vi "Main.vi"(11 "Module Admin":refnum<class "Delacor_lib_QMH_Module Admin.lvclass">) -> ()   [LabVIEW 2018, in "Example.lvlib"]
doc: "This template is based off of the Queued Message Handler design pattern and the Queued Message Handler project template that ships with LabVIEW.\n\nThe main difference is that the queue is private to this module and communication between modules is performed via Broadcast and Request events.\n\nRequest events are wrapped in public API methods and are handled in the Event Handling Loop (EHL) of this VI. Any module can register for Broadcast events sent by this module. The EHL generates messages based on user interface actions.\n\nThe Message Handling Loop (MHL) processes messages generated by the EHL, or by other messages. The messages are string values, so new messages can be added easily to the Message Cases case structure in the MHL. Each message cluster can also provide an optional value for Message Data, which is a variant that can be converted to whatever message-specific data is required.\n_____\nBased on DQMH Project Example 6.0.0.91."
uses:
  Example.lvlib
  <vilib>/Delacor/Delacor QMH/Libraries/Message Queue_class/Delacor_lib_QMH_Message Queue.lvclass
  Module Data--cluster.ctl
  <vilib>/Utility/miscctls.llb/LVPointTypeDef.ctl
  Do Something Argument--cluster.ctl
  Do Something Else Argument--cluster.ctl
  Do Something Else and Wait (Reply Payload)--cluster.ctl
  Do Something Else and Wait for Reply Argument--cluster.ctl
  <vilib>/Utility/error.llb/Error Cluster From Error Code.vi
  <vilib>/ErrorRing/Error Ring.xnode
  <vilib>/Delacor/Delacor QMH/Libraries/Message Queue_class/Delacor_lib_QMH_Enqueue Message (Single).vi
  Stop Argument--cluster.ctl
  <vilib>/Delacor/Delacor QMH/Libraries/Module Admin_class/Delacor_lib_QMH_Module Admin.lvclass
  Get Bitness Info (Reply Payload)--cluster.ctl
  Get Bitness Info Argument--cluster.ctl
panel:
  out "error out":errorcluster
  out "X":dbl
  out "Status":string
  in  "Simulate MHL Error":bool
  in  "Simulate EHL Error":bool
  in  "Do Something Else <Replace Me>":bool
  in  "Do Something <Replace Me>":bool
  # "These controls have associated \"Value Changed\" events configured in the Event Structure on the diagram.\n\nReplace them (and reconfigure the Event Structure) with the controls you need for your application. \n\nOther QMH Modules communicate with this Module via its Public API (wrappers for its Request Events).\n\nThis Module communicates with other Modules via its Broadcast Events.\nAny module that wants to get these messages, just registers for this module's Broadcast events."
  # "This template is for the Delacor Modified Queued Message Handler design pattern.\n\nSee the block diagram for more information on how to use this template."
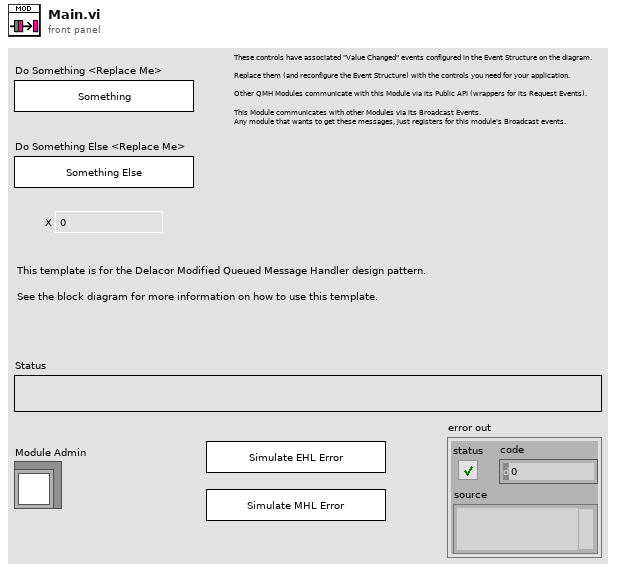
[diagram p1: front panel]
types:
  T1 = typedef "Example.lvlib/Request Events--cluster.ctl" = cluster{"Stop Module":refnum<user-event>, "Do Something":refnum<user-event>, "Do Something Else":refnum<user-event>, "Do Something Else and Wait for Reply":refnum<user-event>, "Show Panel":refnum<user-event>, "Hide Panel":refnum<user-event>, "Get Module Execution Status":refnum<user-event>, "Show Diagram":refnum<user-event>, "Get Bitness Info":refnum<user-event>}
  T2 = typedef "Example.lvlib/Module Data--cluster.ctl" = cluster{"Status":string}
  T3 = typedef "Example.lvlib/Do Something Argument--cluster.ctl" = cluster{"Do Something Msg":string}
  T4 = typedef "Example.lvlib/Do Something Else Argument--cluster.ctl" = cluster{"Do Something Else Msg":string, "X":dbl}
  T5 = typedef "Example.lvlib/Do Something Else and Wait for Reply Argument--cluster.ctl" = cluster{"Do Something Else Msg":string, "X":dbl, "Wait Notifier":refnum<notifier>, "wait for reply":bool}
  T6 = enum32{"invalid lock state", "Not Locked", "Locked (No Password)", "Password-protected"}
  T7 = typedef "Example.lvlib/Stop Argument--cluster.ctl" = cluster{"Origin":string, "Exit via Stop Module Req?":bool, "Wait for Module to stop?":bool}
  T8 = typedef "Example.lvlib/Get Bitness Info Argument--cluster.ctl" = cluster{"Wait Notifier":refnum<notifier>, "wait for reply":bool}
  T9 = typedef "LVPointTypeDef.ctl" = cluster{"Horizontal":i16, "Vertical":i16}
  T10 = enum32{"Invalid", "Standard", "Closed", "Hidden", "Minimized", "Maximized"}
  T11 = typedef "Example.lvlib/Do Something Else and Wait (Reply Payload)--cluster.ctl" = cluster{"Value":dbl, "error":errorcluster}
  T12 = typedef "Example.lvlib/Get Bitness Info (Reply Payload)--cluster.ctl" = cluster{"BitnessInfo":string, "Get Bitness Info_error":errorcluster}
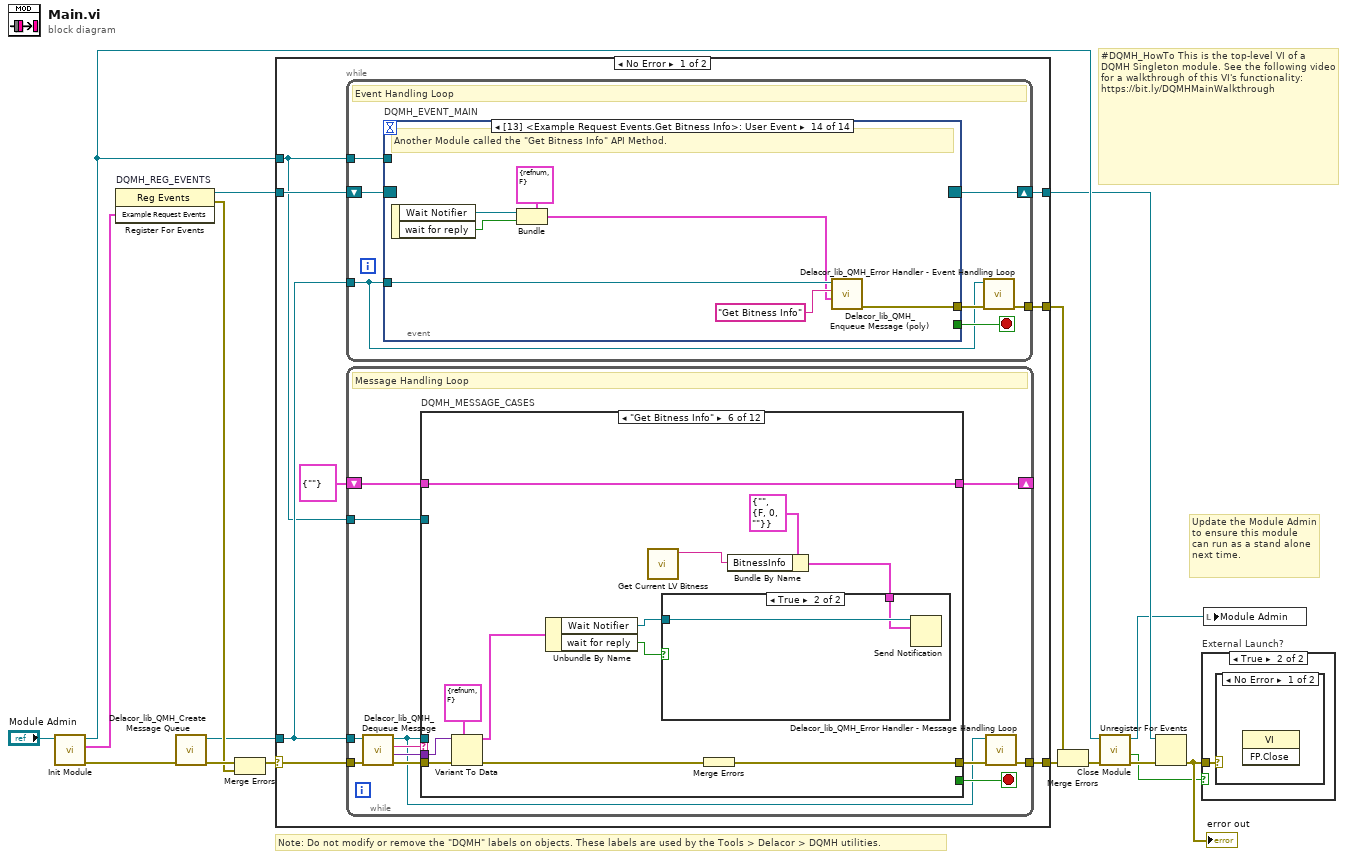
[diagram p0: block diagram]
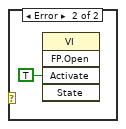
[diagram p3: hidden frame]
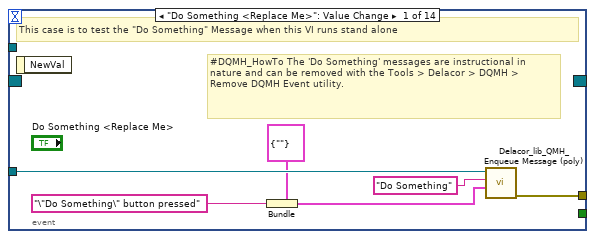
[diagram p4: hidden frame]
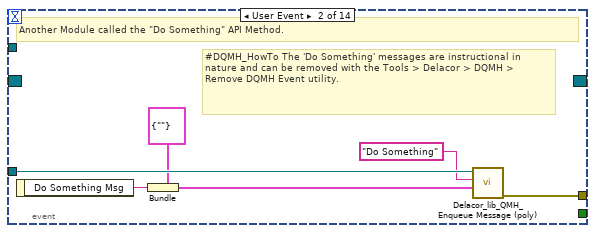
[diagram p5: hidden frame]
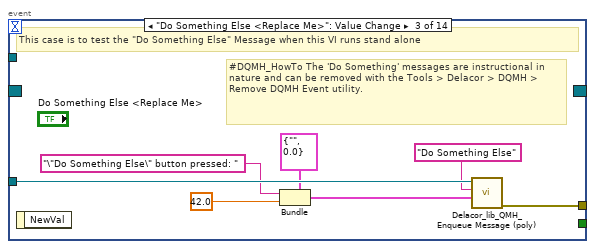
[diagram p6: hidden frame]
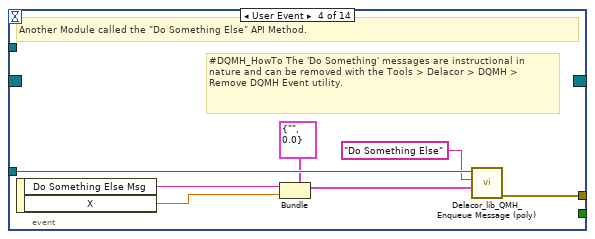
[diagram p7: hidden frame]
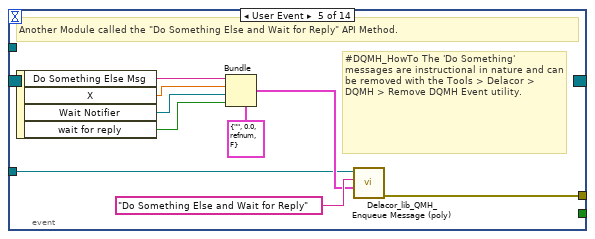
[diagram p8: hidden frame]
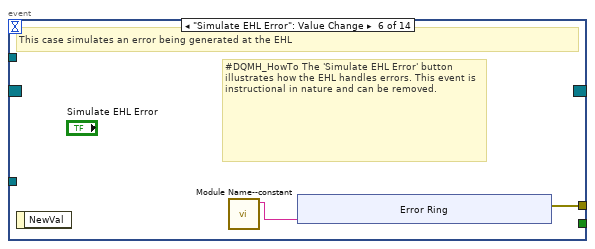
[diagram p9: hidden frame]
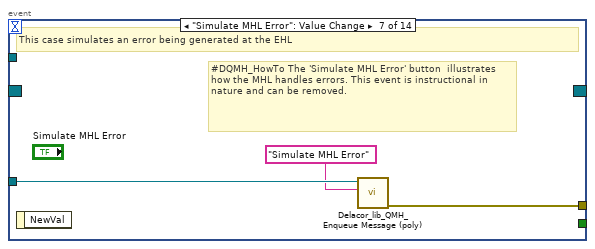
[diagram p10: hidden frame]
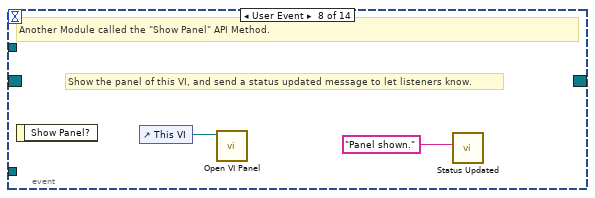
[diagram p11: hidden frame]
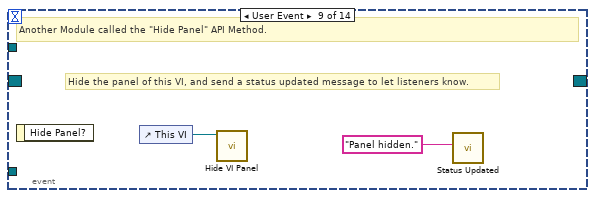
[diagram p12: hidden frame]
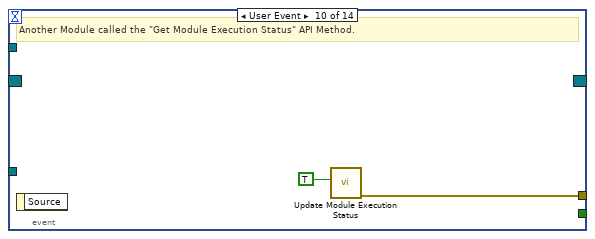
[diagram p13: hidden frame]
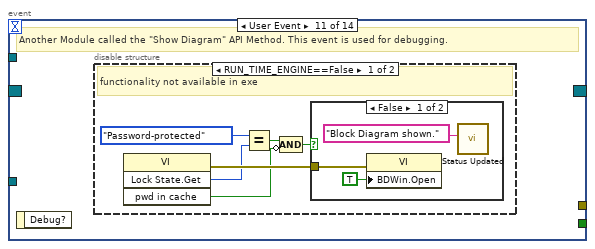
[diagram p14: hidden frame]
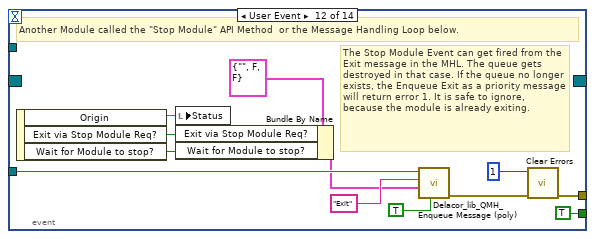
[diagram p17: hidden frame]
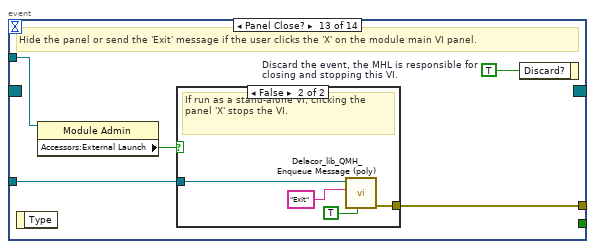
[diagram p18: hidden frame]
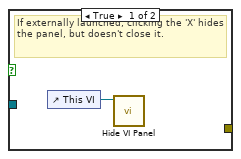
[diagram p19: hidden frame]
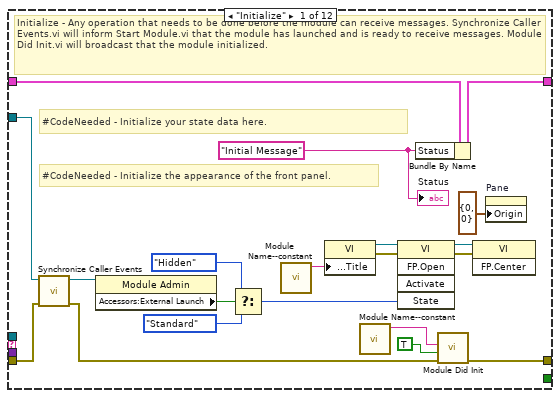
[diagram p20: hidden frame]
diagram:
  # "#DQMH_HowTo This is the top-level VI of a DQMH Singleton module. See the following video for a walkthrough of this VI's functionality: https://bit.ly/DQMHMainWalkthrough"
  # "Note: Do not modify or remove the \"DQMH\" labels on objects. These labels are used by the Tools > Delacor > DQMH utilities."
  # "Update the Module Admin to ensure this module can run as a stand alone next time."
  n1 = call "Init Module.vi"("Singleton Module Admin in"="Module Admin") -> ("error out"=w16:errorcluster, "Example Request Events"=w5:T1, "Singleton Module Admin out"=w8:refnum<class "Delacor_lib_QMH_Module Admin.lvclass">)  [unwired: 8 in]
  n2 = register-events "DQMH_REG_EVENTS"(w5) -> (reference out=w6:refnum<event-registration>, error out=w9:errorcluster)  [unwired: 2 in]
  n3 = call <vilib>:"Delacor_lib_QMH_Create Message Queue.vi"("error in"=w16) -> ("error out"=w11:errorcluster, "Message Queue"=w4:refnum<class "Delacor_lib_QMH_Message Queue.lvclass">)  [unwired: 9 in]
  n4 = Merge Errors(w11, w9) -> (w10:errorcluster)
  n5 = case shown="No Error" w10 {
    selector: w10 -> [w23 w284]
    tunnel: [w25 w283] -> w17
    tunnel: [w22 w289] -> w7
    tunnel: w6 -> [w20 w289]
    tunnel: w4 -> [w19 w282]
    tunnel: [w24 _] -> w14
    tunnel: w8 -> [w18 w285]
    frame No Error {
      n6 = while {
        tunnel: w19 -> [w26]
        shift-right: [w29] -> w22
        shift-left: w20 -> [w30]
        tunnel: [w31] -> w24
        tunnel: w18 -> [w27]
        stop <- w28 stop-if-true
        # "Event Handling Loop"
        n7 = event "DQMH_EVENT_MAIN" shown="[13] <Example Request Events.Get Bitness Info>: User Event" {
          selector: w30 -> [_ _ _ _ _ _ _ _ _ _ _ _ _ _]
          dyn-events: [_ _ _ _ _ _ _ _ _ _ _ _ _ _] -> w29
          timeout: _ -> [_ _ _ _ _ _ _ _ _ _ _ _ _ _]
          tunnel: [_ _ _ _ _ _ _ _ _ _ _ TRUE ("Discard?") _ _] -> w28
          tunnel: w26 -> [w37 w43 w50 w57 w60 _ w78 _ _ _ _ w102 w109 w123]
          tunnel: [w38 w44 w51 w58 w67 w69 w79 _ _ w85 _ w105 w111 w117] -> w32
          tunnel: w27 -> [_ _ _ _ _ _ _ _ _ _ _ _ w108 _]
          event "Do Something <Replace Me>": Value Change {
            # "#DQMH_HowTo The 'Do Something' messages are instructional in nature and can be removed with the Tools > Delacor > DQMH > Remove DQMH Event utility."
            # "This case is to test the \"Do Something\" Message when this VI runs stand alone"
            n8 = event-data() -> ()  [unwired: 1 in, 1 out]
            n9 = Bundle(cluster=T3 {"Do Something Msg"=""} ("Do Something Argument"), "Do Something Msg"="\"Do Something\" button pressed" ("\"Do Something\" button pressed")) -> (w33:T3)
            n10 = call-poly <vilib>:"Delacor_lib_QMH_Enqueue Message (poly).vi"("Message Data"=w33, "Message"="Do Something", "Message Queue in"=w37) -> ("error out"=w38:errorcluster)  [unwired: 7 in, 1 out]
          }
          event User Event {
            # "#DQMH_HowTo The 'Do Something' messages are instructional in nature and can be removed with the Tools > Delacor > DQMH > Remove DQMH Event utility."
            # "Another Module called the \"Do Something\" API Method."
            n11 = event-data() -> ("Do Something Msg"=w40:string)  [unwired: 1 in]
            n12 = Bundle(cluster=T3 {"Do Something Msg"=""} ("Do Something Argument"), "Do Something Msg"=w40) -> (w39:T3)
            n13 = call-poly <vilib>:"Delacor_lib_QMH_Enqueue Message (poly).vi"("Message Data"=w39, "Message"="Do Something", "Message Queue in"=w43) -> ("error out"=w44:errorcluster)  [unwired: 7 in, 1 out]
          }
          event "Do Something Else <Replace Me>": Value Change {
            # "#DQMH_HowTo The 'Do Something' messages are instructional in nature and can be removed with the Tools > Delacor > DQMH > Remove DQMH Event utility."
            # "This case is to test the \"Do Something Else\" Message when this VI runs stand alone"
            n14 = event-data() -> ()  [unwired: 1 in, 1 out]
            n15 = Bundle(cluster=T4 {"Do Something Else Msg"="", "X"=0.0} ("Do Something Else Argument"), "Do Something Else Msg"="\"Do Something Else\" button pressed: " ("\"Do Something Else\" button pressed"), "X"=42.0) -> (w47:T4)
            n16 = call-poly <vilib>:"Delacor_lib_QMH_Enqueue Message (poly).vi"("Message Data"=w47, "Message"="Do Something Else", "Message Queue in"=w50) -> ("error out"=w51:errorcluster)  [unwired: 7 in, 1 out]
          }
          event User Event {
            # "#DQMH_HowTo The 'Do Something' messages are instructional in nature and can be removed with the Tools > Delacor > DQMH > Remove DQMH Event utility."
            # "Another Module called the \"Do Something Else\" API Method."
            n17 = event-data() -> ("Do Something Else Msg"=w53:string, "X"=w52:dbl)  [unwired: 1 in]
            n18 = Bundle(cluster=T4 {"Do Something Else Msg"="", "X"=0.0} ("Do Something Else Argument"), "Do Something Else Msg"=w53, "X"=w52) -> (w54:T4)
            n19 = call-poly <vilib>:"Delacor_lib_QMH_Enqueue Message (poly).vi"("Message Data"=w54, "Message"="Do Something Else", "Message Queue in"=w57) -> ("error out"=w58:errorcluster)  [unwired: 7 in, 1 out]
          }
          event User Event {
            # "#DQMH_HowTo The 'Do Something' messages are instructional in nature and can be removed with the Tools > Delacor > DQMH > Remove DQMH Event utility."
            # "Another Module called the \"Do Something Else and Wait for Reply\" API Method."
            n20 = event-data() -> ("Do Something Else Msg"=w63:string, "X"=w62:dbl, "Wait Notifier"=w61:refnum<notifier>, "wait for reply"=w59:bool)  [unwired: 1 in]
            n21 = Bundle(cluster=T5 {"Do Something Else Msg"="", "X"=0.0, "Wait Notifier"=refnum, "wait for reply"=FALSE} ("Do Something Else and Wait for Reply Argument"), "Do Something Else Msg"=w63, "X"=w62, "Wait Notifier"=w61, "wait for reply"=w59) -> (w64:T5)
            n22 = call-poly <vilib>:"Delacor_lib_QMH_Enqueue Message (poly).vi"("Message Data"=w64, "Message"="Do Something Else and Wait for Reply", "Message Queue in"=w60) -> ("error out"=w67:errorcluster)  [unwired: 7 in, 1 out]
          }
          event "Simulate EHL Error": Value Change {
            # "#DQMH_HowTo The 'Simulate EHL Error' button  illustrates how the EHL handles errors. This event is instructional in nature and can be removed."
            # "This case simulates an error being generated at the EHL"
            n23 = event-data() -> ()  [unwired: 1 in, 1 out]
            n24 = call "Module Name--constant.vi"() -> ("Module Name"=w68:string)  [unwired: 11 in]
            n25 = xnode "Error Ring"("parameter 0"=w68) -> ("error out"=w69:errorcluster)
          }
          event "Simulate MHL Error": Value Change {
            # "#DQMH_HowTo The 'Simulate MHL Error' button  illustrates how the MHL handles errors. This event is instructional in nature and can be removed."
            # "This case simulates an error being generated at the EHL"
            n26 = event-data() -> ()  [unwired: 1 in, 1 out]
            n27 = call-poly <vilib>:"Delacor_lib_QMH_Enqueue Message (poly).vi"("Message"="Simulate MHL Error", "Message Queue in"=w78) -> ("error out"=w79:errorcluster)  [unwired: 8 in, 1 out]
          }
          event User Event {
            # "Show the panel of this VI, and send a status updated message to let listeners know."
            # "Another Module called the \"Show Panel\" API Method."
            n28 = event-data() -> ()  [unwired: 1 in, 1 out]
            n29 = control-ref of="This VI"() -> (w81:refnum<vi>)
            n30 = call "Open VI Panel.vi"("VI"=w81) -> ()  [unwired: 10 in, 1 out]
            n31 = call "Status Updated.vi"("Status"="Panel shown." ("format string")) -> ()  [unwired: 10 in, 1 out]
          }
          event User Event {
            # "Hide the panel of this VI, and send a status updated message to let listeners know."
            # "Another Module called the \"Hide Panel\" API Method."
            n32 = event-data() -> ()  [unwired: 1 in, 1 out]
            n33 = control-ref of="This VI"() -> (w83:refnum<vi>)
            n34 = call "Hide VI Panel.vi"("VI"=w83) -> ()  [unwired: 10 in, 1 out]
            n35 = call "Status Updated.vi"("Status"="Panel hidden." ("format string")) -> ()  [unwired: 10 in, 1 out]
          }
          event User Event {
            # "Another Module called the \"Get Module Execution Status\" API Method."
            n36 = event-data() -> ()  [unwired: 1 in, 1 out]
            n37 = call "Update Module Execution Status.vi"("Running?"=TRUE) -> ("error out"=w85:errorcluster)  [unwired: 10 in]
          }
          event User Event {
            # "Another Module called the \"Show Diagram\" API Method. This event is used for debugging."
            n38 = event-data() -> ()  [unwired: 1 in, 1 out]
            n39 = disable-structure shown="RUN_TIME_ENGINE==False" {
              frame condition #0 (active) {
                # "functionality not available in exe"
                n40 = invoke class="VI" method="Lock State.Get"() -> (error out=w91:errorcluster, "Get Lock State"=w90:T6, "pwd in cache"=w87:bool)  [unwired: 4 in, 1 out]
                n41 = Equal?(x=T6."Password-protected", y=w90) -> (x = y?=w88:bool)
                n42 = Compound Arithmetic op=AND(w88, invert w87) -> (w86:bool)
                n43 = case shown="False" w86 {
                  tunnel: w91 -> [w94 _]
                  frame False {
                    n44 = property class="VI"(error in=w94, "BDWin.Open"=TRUE ("Block Diagram Window:Open")) -> ()  [unwired: 1 in, 2 out]
                    n45 = call "Status Updated.vi"("Status"="Block Diagram shown." ("format string")) -> ()  [unwired: 10 in, 1 out]
                  }
                  frame True {
                    # "Password-protected VI, and the password is not in the cache. Do not show the diagram."
                  }
                }
              }
              frame condition #1 {
              }
            }
          }
          event User Event {
            # "The Stop Module Event can get fired from the Exit message in the MHL. The queue gets destroyed in that case. If the queue no longer exists, the Enqueue Exit as a priority message will return error 1. It is safe to ignore, because the module is already exiting."
            # "Another Module called the \"Stop Module\" API Method  or the Message Handling Loop below."
            n46 = event-data() -> ("Origin"=w101:string, "Exit via Stop Module Req?"=w97:bool, "Wait for Module to stop?"=w96:bool)  [unwired: 1 in]
            n47 = local write "Status"(w101) -> ()
            n48 = Bundle By Name(cluster=T7 {"Origin"="", "Exit via Stop Module Req?"=FALSE, "Wait for Module to stop?"=FALSE} ("Stop Argument"), "Exit via Stop Module Req?"=w97, "Wait for Module to stop?"=w96) -> (w95:T7)
            n49 = call-poly <vilib>:"Delacor_lib_QMH_Enqueue Message (poly).vi"("Priority Message? (F)"=TRUE, "Message Data"=w95, "Message"="Exit", "Message Queue in"=w102) -> ("error out"=w106:errorcluster)  [unwired: 6 in, 1 out]
            n50 = call <vilib>:"Clear Errors.vi"("error in (no error)"=w106, "specific error code to clear (0: all)"=1) -> ("error out"=w105:errorcluster)  [unwired: 4 in, 1 out]
          }
          event Panel Close? {
            w110 = TRUE  # Discard the event, the MHL is responsible for closing and stopping this VI.
            # "Hide the panel or send the 'Exit' message if the user clicks the 'X' on the module main VI panel."
            n51 = event-data() -> ()  [unwired: 1 in, 1 out]
            n52 = property class="Module Admin"(reference=w108) -> ("Accessors:External Launch"=w107:bool)  [unwired: 1 in, 2 out]
            n53 = case shown="False" w107 {
              tunnel: w109 -> [_ w115]
              tunnel: [_ w116] -> w111
              frame True {
                # "If externally launched, clicking the 'X' hides the panel, but doesn't close it."
                n54 = control-ref of="This VI"() -> (w112:refnum<vi>)
                n55 = call "Hide VI Panel.vi"("VI"=w112) -> ()  [unwired: 10 in, 1 out]
              }
              frame False {
                # "If run as a stand-alone VI, clicking the panel 'X' stops the VI."
                n56 = call-poly <vilib>:"Delacor_lib_QMH_Enqueue Message (poly).vi"("Priority Message? (F)"=TRUE, "Message"="Exit", "Message Queue in"=w115) -> ("error out"=w116:errorcluster)  [unwired: 7 in, 1 out]
              }
            }
            n57 = event-data("Discard?"=w110) -> ()  [unwired: 1 in, 1 out]
          }
          event User Event {
            # "Another Module called the \"Get Bitness Info\" API Method."
            n58 = event-data() -> ("Wait Notifier"=w119:refnum<notifier>, "wait for reply"=w118:bool)  [unwired: 1 in]
            n59 = Bundle(cluster=T8 {"Wait Notifier"=refnum, "wait for reply"=FALSE} ("Get Bitness Info Argument"), "Wait Notifier"=w119, "wait for reply"=w118) -> (w120:T8)
            n60 = call-poly <vilib>:"Delacor_lib_QMH_Enqueue Message (poly).vi"("Message Data"=w120, "Message"="Get Bitness Info", "Message Queue in"=w123) -> ("error out"=w117:errorcluster)  [unwired: 7 in, 1 out]
          }
        }
        n61 = call-dynamic "Delacor_lib_QMH_Error Handler - Event Handling Loop.vi"("error in"=w32, "Message Queue in"=w26) -> ("dup error in"=w31:errorcluster)  [unwired: 8 in, 1 out]
      }
      n62 = while {
        tunnel: w19 -> [w126]
        shift-right: [w130] -> _
        shift-left: T2 {"Status"=""} ("Data Cluster") -> [w131]
        tunnel: w23 -> [w134]
        tunnel: [w132] -> w25
        tunnel: w18 -> [w124]
        stop <- w129 stop-if-true
        # "Message Handling Loop"
        n63 = call-dynamic "Delacor_lib_QMH_Dequeue Message.vi"("error in"=w134, "Message Queue in"=w126) -> ("error out"=w133:errorcluster, "Message Data"=w127:variant, "Message"=w128:string, "Message Queue out"=w125:refnum<class "Delacor_lib_QMH_Message Queue.lvclass">)  [unwired: 6 in]
        n64 = case "DQMH_MESSAGE_CASES" shown="\"Get Bitness Info\"" w128 {
          selector: w128 -> [_ _ _ _ _ _ _ _ _ _ _ w269]
          tunnel: w125 -> [_ _ _ _ _ _ _ _ _ w239 w261 _]
          tunnel: w133 -> [w153 w157 w165 w174 w193 w217 w222 w224 w229 w246 w267 w271]
          tunnel: [w151 w157 w163 w173 w192 w207 w221 w224 w228 w242 w264 w272] -> w135
          tunnel: w131 -> [w142 w156 w162 w172 w190 w216 w220 w223 w226 w241 w260 w270]
          tunnel: [w141 w156 w162 w172 w190 w216 w220 w223 w226 w241 w260 w270] -> w130
          tunnel: [_ _ _ _ _ _ _ _ _ _ w259 _] -> w129
          tunnel: w127 -> [_ _ w161 w169 w187 w214 _ _ _ w240 w258 _]
          tunnel: w124 -> [w143 _ _ _ _ _ _ _ _ w238 w253 _]
          frame "Initialize" {
            w137 = "Initial Message" ("Initial Message")
            # "#CodeNeeded - Initialize the appearance of the front panel."
            # "#CodeNeeded - Initialize your state data here."
            # "Initialize - Any operation that needs to be done before the module can receive messages. Synchronize Caller Events.vi will inform Start Module.vi that the module has launched and is ready to receive messages. Module Did Init.vi will broadcast that the module initialized."
            n65 = call "Synchronize Caller Events.vi"("error in (no error)"=w153, "Singleton Module Admin in"=w143) -> ("error out"=w152:errorcluster, "Singleton Module Admin out"=w138:refnum<class "Delacor_lib_QMH_Module Admin.lvclass">)  [unwired: 8 in]
            n66 = property class="Module Admin"(reference=w138) -> ("Accessors:External Launch"=w147:bool)  [unwired: 1 in, 2 out]
            n67 = Select(t=T10."Hidden" ("State"), s=w147, f=T10."Standard" ("State")) -> (s? t:f=w144:T10)
            n68 = call "Module Name--constant.vi"() -> ("Module Name"=w150:string)  [unwired: 11 in]
            n69 = property class="VI"("Front Panel.Title"=w150) -> (reference out=w149:refnum<vi>, error out=w155:errorcluster)  [unwired: 2 in]
            n70 = call "Module Name--constant.vi"() -> ("Module Name"=w139:string)  [unwired: 11 in]
            n71 = invoke class="VI" method="FP.Open"(reference=w149, error in=w155, "State"=w144) -> (reference out=w148:refnum<vi>, error out=w154:errorcluster)  [unwired: 2 in, 3 out]
            n72 = Bundle By Name(cluster=w142, "Status"=w137) -> (w141:T2)
            n73 = call "Module Did Init.vi"("error in (no error)"=w152, "Initialized?"=TRUE, "Origin"=w139) -> ("error out"=w151:errorcluster)  [unwired: 8 in]
            n74 = invoke class="VI" method="FP.Center"(reference=w148, error in=w154) -> ()  [unwired: 1 in, 3 out]
            n75 = property on="Pane" class="Pane"("Origin"=T9 {"Horizontal"=0, "Vertical"=0}) -> ()  [unwired: 2 in, 2 out]
            "Status" <- w137
          }
          frame "---Module Specific---" {
            # "Separator -- The following cases handle messages specific to this Module."
          }
          frame "Do Something" {
            # "#DQMH_HowTo The 'Do Something' messages are instructional in nature and can be removed with the Tools > Delacor > DQMH > Remove DQMH Event utility."
            # "Do Something - Replace this message with functionality for your own application. Note that this message also fires the \"Did Something\" broadcast event."
            n76 = Variant To Data(error in=w165, type=T3 {"Do Something Msg"=""} ("Do Something Argument"), Variant=w161) -> (data=w160:T3, error out=w164:errorcluster)
            n77 = Unbundle By Name(w160) -> ("Do Something Msg"=w158:string)
            n78 = call "Did Something.vi"("error in (no error)"=w164, "Did Something Msg"=w158) -> ("error out"=w163:errorcluster)  [unwired: 9 in]
            n79 = local write "Status"(w158) -> ()
            n80 = call "Status Updated.vi"("Status"=w158) -> ()  [unwired: 10 in, 1 out]
          }
          frame "Do Something Else" {
            # "#DQMH_HowTo The 'Do Something' messages are instructional in nature and can be removed with the Tools > Delacor > DQMH > Remove DQMH Event utility."
            # "Do Something Else - Replace this message with functionality for your own application."
            n81 = Variant To Data(error in=w174, type=T4 {"Do Something Else Msg"="", "X"=0.0} ("Do Something Else Argument"), Variant=w169) -> (data=w170:T4, error out=w173:errorcluster)
            n82 = Unbundle By Name(w170) -> ("Do Something Else Msg"=w168:string, "X"=w167:dbl)
            "X" <- w167
            n83 = Format Into String(initial string=w168, w167) -> (resulting string=w166:string)  [unwired: 2 in, 1 out]
            n84 = local write "Status"(w166) -> ()
            n85 = call "Status Updated.vi"("Status"=w166) -> ()  [unwired: 10 in, 1 out]
          }
          frame "Do Something Else and Wait for Reply" {
            w182 = "X(%.2f)+Offset(%.2f)=%.2f"  # status message format string
            # "#DQMH_HowTo The 'Do Something' messages are instructional in nature and can be removed."
            # "Send back X with a random offset"
            # "Do Something Else and Wait for Reply - Replace this message with functionality for your own application. Note that this message must fire a notifier to let callers know it has finished execution, and it returns an error if the 'Value' is negative."
            n86 = Random Number (0-1)() -> (number: 0 to 1=w184:dbl)
            n87 = Variant To Data(error in=w193, type=T5 {"Do Something Else Msg"="", "X"=0.0, "Wait Notifier"=refnum, "wait for reply"=FALSE} ("Do Something Else and Wait for Reply Argument"), Variant=w187) -> (data=w188:T5, error out=w191:errorcluster)
            n88 = Unbundle By Name(w188) -> ("Wait Notifier"=w175:refnum<notifier>, "Do Something Else Msg"=w186:string, "X"=w183:dbl, "wait for reply"=w179:bool)
            n89 = Add(x=w184, y=w183) -> (x+y=w178:dbl)
            n90 = local write "X"(w183) -> ()
            n91 = Less Than 0?(x=w178) -> (x < 0?=w181:bool)
            n92 = Format Into String(format string=w182, initial string=w186, w183, w184, w178) -> (resulting string=w180:string)  [unwired: 1 in, 1 out]
            n93 = case shown="True" w181 {
              tunnel: [_ w200] -> w176
              frame False {
              }
              frame True {
                n94 = xnode "Error Ring"() -> ("error out"=w200:errorcluster)
              }
            }
            n95 = Bundle By Name(cluster=T11 {"Value"=0.0, "error"={"status"=FALSE, "code"=0, "source"=""}} ("notification"), "error"=w176, "Value"=w178) -> (w177:T11)
            n96 = local write "Status"(w180) -> ()
            n97 = call "Status Updated.vi"("Status"=w180) -> ()  [unwired: 10 in, 1 out]
            n98 = case shown="True" w179 {
              tunnel: w177 -> [_ w196]
              tunnel: w175 -> [_ w195]
              frame False {
              }
              frame True {
                # "Simulate an operation that requires a wait."
                n99 = flat-sequence {
                  tunnel: w196 -> [w199]
                  tunnel: w195 -> [w198]
                  tunnel: w194 -> [_]
                  frame #0 {
                    n100 = Send Notification(notification=w199, notifier=w198) -> ()  [unwired: 1 in, 2 out]
                  }
                }
                n101 = Wait (ms)(milliseconds to wait=u32 1000) -> (millisecond timer value=w194:u32)
              }
            }
            n102 = Merge Errors(w191, w176) -> (w192:errorcluster)
          }
          frame "Get Bitness Info" {
            n103 = Variant To Data(error in=w217, type=T8 {"Wait Notifier"=refnum, "wait for reply"=FALSE} ("Get Bitness Info Argument"), Variant=w214) -> (data=w212:T8, error out=w215:errorcluster)
            n104 = Unbundle By Name(w212) -> ("Wait Notifier"=w211:refnum<notifier>, "wait for reply"=w210:bool)
            n105 = call <vilib>:"Get Current LV Bitness.vi"() -> ("bitness"=w206:string)  [unwired: 11 in]
            n106 = Merge Errors(w215) -> (w207:errorcluster)
            n107 = Bundle By Name(cluster=T12 {"BitnessInfo"="", "Get Bitness Info_error"={"status"=FALSE, "code"=0, "source"=""}} ("Get Bitness Info (Reply Payload)"), "BitnessInfo"=w206) -> (w209:T12)
            n108 = case shown="True" w210 {
              tunnel: w211 -> [_ w219]
              tunnel: w209 -> [_ w218]
              frame False {
              }
              frame True {
                n109 = Send Notification(notification=w218, notifier=w219) -> ()  [unwired: 1 in, 2 out]
              }
            }
          }
          frame "---Copy This Frame---" {
            # "Duplicate this frame when creating new messages.  Change this comment in the duplicated frame to describe this message."
            n110 = Merge Errors(w222) -> (w221:errorcluster)
          }
          frame "---Exit and Error Handling---" {
            # "Separator - The following cases handle errors and exit messages."
          }
          frame "Simulate MHL Error" {
            # "#DQMH_HowTo The 'Simulate MHL Error' button  illustrates how the MHL handles errors. This event is instructional in nature and can be removed."
            # "Simulate an error occurring at the MHL"
            n111 = call "Module Name--constant.vi"() -> ("Module Name"=w225:string)  [unwired: 11 in]
            n112 = xnode "Error Ring"("parameter 0"=w225) -> ("error out"=w227:errorcluster)
            n113 = Merge Errors(w229, w227) -> (w228:errorcluster)
          }
          frame "Error" {
            # "#CodeRecommended - If you ever change the name of this \"Error\" message, you'll need to update the name in the Check Loop Error.vi as well."
            # "#CodeRecommended - If the module is running in standalone mode (External Launch = FALSE), this code will pop up an error dialog and call the 'Exit' message if an error occurs. Add more fine-grained error handling here."
            # "Error - Check the error message data and respond accordingly. This message is sent by the \"Error Handler\" VIs at the end of each loop in this application."
            n114 = property class="Module Admin"(reference=w238) -> ("Accessors:External Launch"=w237:bool)  [unwired: 1 in, 2 out]
            n115 = Variant To Data(error in=w246, type=errorcluster {"status"=FALSE, "code"=0, "source"=""} ("error constant"), Variant=w240) -> (data=w247:errorcluster, error out=w244:errorcluster)
            n116 = call "Error Reported.vi"("Error"=w247) -> ()  [unwired: 10 in, 1 out]
            n117 = case shown="False" w237 {
              tunnel: [w252 _] -> w243
              tunnel: w239 -> [w250 _]
              tunnel: w247 -> [w251 _]
              frame False {
                # "If the module is running standalone, then pop up an error dialog and call the \"Exit\" message."
                n118 = call <vilib>:"Simple Error Handler.vi"("error in (no error)"=w251) -> ()  [unwired: 4 in, 5 out]
                n119 = call-poly <vilib>:"Delacor_lib_QMH_Enqueue Message (poly).vi"("Priority Message? (F)"=TRUE, "Message"="Exit", "Message Queue in"=w250) -> ("error out"=w252:errorcluster)  [unwired: 7 in, 1 out]
              }
              frame True {
                # "If the module was launched externally, calling the Error Reported broadcast VI is the only action performed by the \"Error\" message. The module's caller can then process the error appropriately."
              }
            }
            n120 = Merge Errors(w244, w243) -> (w242:errorcluster)
            n121 = local write "error out"(w242) -> ()
          }
          frame "Exit" {
            w257 = 91  # 91: not all Exit messages will have an argument
            w259 = TRUE  # Stop the VI
            # "Release the message queue reference"
            # "#CodeNeeded - Add any required cleanup code here"
            # "Exit - Exit the application."
            n122 = Variant To Data(error in=w267, type=T7 {"Origin"="", "Exit via Stop Module Req?"=FALSE, "Wait for Module to stop?"=FALSE} ("Stop Argument"), Variant=w258) -> (data=w255:T7, error out=w263:errorcluster)
            n123 = call <vilib>:"Clear Errors.vi"("error in (no error)"=w263, "specific error code to clear (0: all)"=w257) -> ("error out"=w266:errorcluster)  [unwired: 4 in, 1 out]
            n124 = control-ref of="This VI"() -> (w254:refnum<vi>)
            n125 = call-dynamic "Delacor_lib_QMH_Release Message Queue.vi"("error in"=w266, "Message Queue"=w261) -> ("error out"=w265:errorcluster)  [unwired: 9 in]
            n126 = call "Handle Exit.vi"("Stop Argument"=w255, "Admin in"=w253, "VI reference"=w254) -> ("error out"=w262:errorcluster)  [unwired: 7 in, 1 out]
            n127 = Merge Errors(w265, w262) -> (w264:errorcluster)
          }
          frame Default {
            # "'Default' case only runs if there is a message that isn't defined in any of the other cases.  Output a programming error."
            n128 = call "Module Name--constant.vi"() -> ("Module Name"=w268:string)  [unwired: 11 in]
            n129 = xnode "Error Ring"("parameter 0"=w269, "parameter 1"=w268) -> ("error out"=w273:errorcluster)
            n130 = Merge Errors(w271, w273) -> (w272:errorcluster)
          }
        }
        n131 = call-dynamic "Delacor_lib_QMH_Error Handler - Message Handling Loop.vi"("error in"=w135, "Message Queue in"=w125) -> ("dup error in"=w132:errorcluster)  [unwired: 8 in, 1 out]
      }
    }
    frame Error {
      # "Synchronize Caller Events.vi will inform Start Module.vi that the module has launched and will let the code calling Start Module.vi register for broadcasts and would permit the caller receive the broadcast that an error occurred at launch time."
      n132 = call-dynamic "Delacor_lib_QMH_Release Message Queue.vi"("error in"=w284, "Message Queue"=w282) -> ("error out"=w283:errorcluster)  [unwired: 9 in]
      n133 = call "Synchronize Caller Events.vi"("Singleton Module Admin in"=w285) -> ("error out"=w290:errorcluster)  [unwired: 9 in, 1 out]
      n134 = call "Module Name--constant.vi"() -> ("Module Name"=w288:string)  [unwired: 11 in]
      n135 = Format Into String(format string="An error occurred during initialization. %s is no longer running.", w288) -> (resulting string=w286:string)  [unwired: 2 in, 1 out]
      n136 = Merge Errors(w283, w290) -> (w291:errorcluster)
      n137 = call "Error Reported.vi"("Additional Information"=w286, "Error"=w291) -> ()  [unwired: 9 in, 1 out]
    }
  }
  n138 = Merge Errors(w14, w17) -> (w13:errorcluster)
  n139 = call "Close Module.vi"("error in (no error)"=w13, "Module Admin in"=w8) -> ("error out"=w15:errorcluster, "External Launch"=w1:bool, "Module Admin out"=w2:refnum<class "Delacor_lib_QMH_Module Admin.lvclass">)  [unwired: 7 in]
  n140 = Unregister For Events(event registration refnum=w7, error in=w15) -> (error out=w12:errorcluster)
  "error out" <- w12
  n141 = case "External Launch?" shown="True" w1 {
    tunnel: w12 -> [_ w292]
    frame False {
    }
    frame True {
      n142 = case shown="No Error" w292 {
        frame No Error {
          n143 = invoke class="VI" method="FP.Close"() -> ()  [unwired: 3 in, 3 out]
        }
        frame Error {
          n144 = invoke class="VI" method="FP.Open"("Activate"=TRUE ("Activate?")) -> ()  [unwired: 4 in, 5 out]
        }
      }
    }
  }
  n145 = local write "Module Admin"(w2) -> ()
